vi "Half-H.vi"(8 "error in (no error)":errorcluster, 11 "Node Ptr":T8 format="%.0x") -> (0 "error out":errorcluster)   [LabVIEW 2016, in "DCM System Explorer.lvlib"]
uses:
  DCM System Explorer.lvlib
  <vilib>/NI Veristand/Custom Device API/Custom Device Item Ref.ctl
  <vilib>/Powertrain Controls/Device Drivers/DCM/HH/RT/Setup.ctl
  <vilib>/Powertrain Controls/Device Drivers/DCM/HH/FPGA/Mode.ctl
  <vilib>/Powertrain Controls/Device Drivers/DCM/Rev0/FPGA/Digital Channel.ctl
  <vilib>/Powertrain Controls/Device Drivers/DCM/HH/RT/Angle Control.ctl
  <vilib>/Powertrain Controls/Device Drivers/DCM/HH/RT/Config.ctl
  <vilib>/Powertrain Controls/Device Drivers/DCM/HH/RT/Mode.ctl
  <vilib>/Powertrain Controls/Device Drivers/DCM/HH/RT/ISeq.ctl
  Shared/DCM Properties.vi
  <vilib>/NI Veristand/Custom Device API/Get Item Property (String Array).vi
  Shared/DCM Constants and GUIDs.vi
  <vilib>/NI Veristand/Custom Device API/Set Item Property (String Array).vi
  <vilib>/NI VeriStand/Custom Device API/Custom Device API.lvlib
  DCM Shared.lvlib
  <vilib>/Powertrain Controls/Device Drivers/DCM/HH/RT/DCM - RT - HH.lvlib
  <vilib>/Powertrain Controls/Device Drivers/DCM/Rev0/FPGA/DCM - FPGA.lvlib
  <vilib>/Powertrain Controls/Device Drivers/DCM/HH/FPGA/DCM - FPGA - HH.lvlib
panel:
  in  "Channel Name":string
  in  "Channel Names":string[](array[string])=["", "", "", "", "", "", "", "", "", "", "", ""]
  in  "_Refresh":bool
  in  "_CommandElement":T1={"Mode"=enum."Off", "Digital Input"=enum."Unused", "Polarity"=FALSE, "Frequency [Hz]"=0.0, "Duty Cycle [%]"=0.0, "TDC Offset [CAD]"=0.0, "Window Start [DBTDC]"=0.0, "Window End [DBTDC]"=0.0, "Angles"=[{"Enable"=FALSE, "Location [DBTDC]"=0.0, "Duration [s]"=0.0}, {"Enable"=FALSE, "Location [DBTDC]"=0.0, "Duration [s]"=0.0}, {"Enable"=FALSE, "Location [DBTDC]"=0.0, "Duration [s]"=0.0}, {"Enable"=FALSE, "Location [DBTDC]"=0.0, "Duration [s]"=0.0}], "Skip Fire"=FALSE, "Skip Fire Index"=0} caption="Command Setup" {"Skip Fire Index" max=7; "Angles"."Duration [s]" format="%#_3p"; "Frequency [Hz]" format="%#_3p"}
  in  "_ConfigElement":T5 caption="Channel Configuration" {"ISeq"."Duration [s]" min=0 max=26 format="%#_3p"; "ISeq"."Lower [A]" min=0 max=8 format="%#_3p"; "ISeq"."Upper [A]" min=0 max=8 format="%#_3p"}
  in  "_HH Channels":i32[](listbox) caption="Half-H Channel Summary"
  in  "_Save Changes?":bool
  in  "Command":T1[](array[typedef])=[{"Mode"=enum."Off", "Digital Input"=enum."Unused", "Polarity"=FALSE, "Frequency [Hz]"=0.0, "Duty Cycle [%]"=0.0, "TDC Offset [CAD]"=0.0, "Window Start [DBTDC]"=0.0, "Window End [DBTDC]"=0.0, "Angles"=[{"Enable"=FALSE, "Location [DBTDC]"=0.0, "Duration [s]"=0.0}, {"Enable"=FALSE, "Location [DBTDC]"=0.0, "Duration [s]"=0.0}, {"Enable"=FALSE, "Location [DBTDC]"=0.0, "Duration [s]"=0.0}, {"Enable"=FALSE, "Location [DBTDC]"=0.0, "Duration [s]"=0.0}], "Skip Fire"=FALSE, "Skip Fire Index"=0}, {"Mode"=enum."Off", "Digital Input"=enum."Unused", "Polarity"=FALSE, "Frequency [Hz]"=0.0, "Duty Cycle [%]"=0.0, "TDC Offset [CAD]"=0.0, "Window Start [DBTDC]"=0.0, "Window End [DBTDC]"=0.0, "Angles"=[{"Enable"=FALSE, "Location [DBTDC]"=0.0, "Duration [s]"=0.0}, {"Enable"=FALSE, "Location [DBTDC]"=0.0, "Duration [s]"=0.0}, {"Enable"=FALSE, "Location [DBTDC]"=0.0, "Duration [s]"=0.0}, {"Enable"=FALSE, "Location [DBTDC]"=0.0, "Duration [s]"=0.0}], "Skip Fire"=FALSE, "Skip Fire Index"=0}, {"Mode"=enum."Off", "Digital Input"=enum."Unused", "Polarity"=FALSE, "Frequency [Hz]"=0.0, "Duty Cycle [%]"=0.0, "TDC Offset [CAD]"=0.0, "Window Start [DBTDC]"=0.0, "Window End [DBTDC]"=0.0, "Angles"=[{"Enable"=FALSE, "Location [DBTDC]"=0.0, "Duration [s]"=0.0}, {"Enable"=FALSE, "Location [DBTDC]"=0.0, "Duration [s]"=0.0}, {"Enable"=FALSE, "Location [DBTDC]"=0.0, "Duration [s]"=0.0}, {"Enable"=FALSE, "Location [DBTDC]"=0.0, "Duration [s]"=0.0}], "Skip Fire"=FALSE, "Skip Fire Index"=0}, {"Mode"=enum."Off", "Digital Input"=enum."Unused", "Polarity"=FALSE, "Frequency [Hz]"=0.0, "Duty Cycle [%]"=0.0, "TDC Offset [CAD]"=0.0, "Window Start [DBTDC]"=0.0, "Window End [DBTDC]"=0.0, "Angles"=[{"Enable"=FALSE, "Location [DBTDC]"=0.0, "Duration [s]"=0.0}, {"Enable"=FALSE, "Location [DBTDC]"=0.0, "Duration [s]"=0.0}, {"Enable"=FALSE, "Location [DBTDC]"=0.0, "Duration [s]"=0.0}, {"Enable"=FALSE, "Location [DBTDC]"=0.0, "Duration [s]"=0.0}], "Skip Fire"=FALSE, "Skip Fire Index"=0}, {"Mode"=enum."Off", "Digital Input"=enum."Unused", "Polarity"=FALSE, "Frequency [Hz]"=0.0, "Duty Cycle [%]"=0.0, "TDC Offset [CAD]"=0.0, "Window Start [DBTDC]"=0.0, "Window End [DBTDC]"=0.0, "Angles"=[{"Enable"=FALSE, "Location [DBTDC]"=0.0, "Duration [s]"=0.0}, {"Enable"=FALSE, "Location [DBTDC]"=0.0, "Duration [s]"=0.0}, {"Enable"=FALSE, "Location [DBTDC]"=0.0, "Duration [s]"=0.0}, {"Enable"=FALSE, "Location [DBTDC]"=0.0, "Duration [s]"=0.0}], "Skip Fire"=FALSE, "Skip Fire Index"=0}, {"Mode"=enum."Off", "Digital Input"=enum."Unused", "Polarity"=FALSE, "Frequency [Hz]"=0.0, "Duty Cycle [%]"=0.0, "TDC Offset [CAD]"=0.0, "Window Start [DBTDC]"=0.0, "Window End [DBTDC]"=0.0, "Angles"=[{"Enable"=FALSE, "Location [DBTDC]"=0.0, "Duration [s]"=0.0}, {"Enable"=FALSE, "Location [DBTDC]"=0.0, "Duration [s]"=0.0}, {"Enable"=FALSE, "Location [DBTDC]"=0.0, "Duration [s]"=0.0}, {"Enable"=FALSE, "Location [DBTDC]"=0.0, "Duration [s]"=0.0}], "Skip Fire"=FALSE, "Skip Fire Index"=0}, {"Mode"=enum."Off", "Digital Input"=enum."Unused", "Polarity"=FALSE, "Frequency [Hz]"=0.0, "Duty Cycle [%]"=0.0, "TDC Offset [CAD]"=0.0, "Window Start [DBTDC]"=0.0, "Window End [DBTDC]"=0.0, "Angles"=[{"Enable"=FALSE, "Location [DBTDC]"=0.0, "Duration [s]"=0.0}, {"Enable"=FALSE, "Location [DBTDC]"=0.0, "Duration [s]"=0.0}, {"Enable"=FALSE, "Location [DBTDC]"=0.0, "Duration [s]"=0.0}, {"Enable"=FALSE, "Location [DBTDC]"=0.0, "Duration [s]"=0.0}], "Skip Fire"=FALSE, "Skip Fire Index"=0}, {"Mode"=enum."Off", "Digital Input"=enum."Unused", "Polarity"=FALSE, "Frequency [Hz]"=0.0, "Duty Cycle [%]"=0.0, "TDC Offset [CAD]"=0.0, "Window Start [DBTDC]"=0.0, "Window End [DBTDC]"=0.0, "Angles"=[{"Enable"=FALSE, "Location [DBTDC]"=0.0, "Duration [s]"=0.0}, {"Enable"=FALSE, "Location [DBTDC]"=0.0, "Duration [s]"=0.0}, {"Enable"=FALSE, "Location [DBTDC]"=0.0, "Duration [s]"=0.0}, {"Enable"=FALSE, "Location [DBTDC]"=0.0, "Duration [s]"=0.0}], "Skip Fire"=FALSE, "Skip Fire Index"=0}] {"Skip Fire Index" max=7; "Angles"."Duration [s]" format="%#_3p"; "Frequency [Hz]" format="%#_3p"}
  in  "Config":T5[](array[typedef])=[{"Mode"=enum."Off", "IO Lock State"=FALSE, "Phase 1 FP"=FALSE, "Fault Clear"=FALSE, "ISeq"=[]}, {"Mode"=enum."Off", "IO Lock State"=FALSE, "Phase 1 FP"=FALSE, "Fault Clear"=FALSE, "ISeq"=[]}, {"Mode"=enum."Off", "IO Lock State"=FALSE, "Phase 1 FP"=FALSE, "Fault Clear"=FALSE, "ISeq"=[]}, {"Mode"=enum."Off", "IO Lock State"=FALSE, "Phase 1 FP"=FALSE, "Fault Clear"=FALSE, "ISeq"=[]}, {"Mode"=enum."Off", "IO Lock State"=FALSE, "Phase 1 FP"=FALSE, "Fault Clear"=FALSE, "ISeq"=[]}, {"Mode"=enum."Off", "IO Lock State"=FALSE, "Phase 1 FP"=FALSE, "Fault Clear"=FALSE, "ISeq"=[]}, {"Mode"=enum."Off", "IO Lock State"=FALSE, "Phase 1 FP"=FALSE, "Fault Clear"=FALSE, "ISeq"=[]}, {"Mode"=enum."Off", "IO Lock State"=FALSE, "Phase 1 FP"=FALSE, "Fault Clear"=FALSE, "ISeq"=[]}] {"ISeq"."Duration [s]" min=0 max=26 format="%#_3p"; "ISeq"."Lower [A]" min=0 max=8 format="%#_3p"; "ISeq"."Upper [A]" min=0 max=8 format="%#_3p"}
  in  "Header":cluster{"Section Name":string}={"Section Name"="Half-H Drive Initial Settings"}
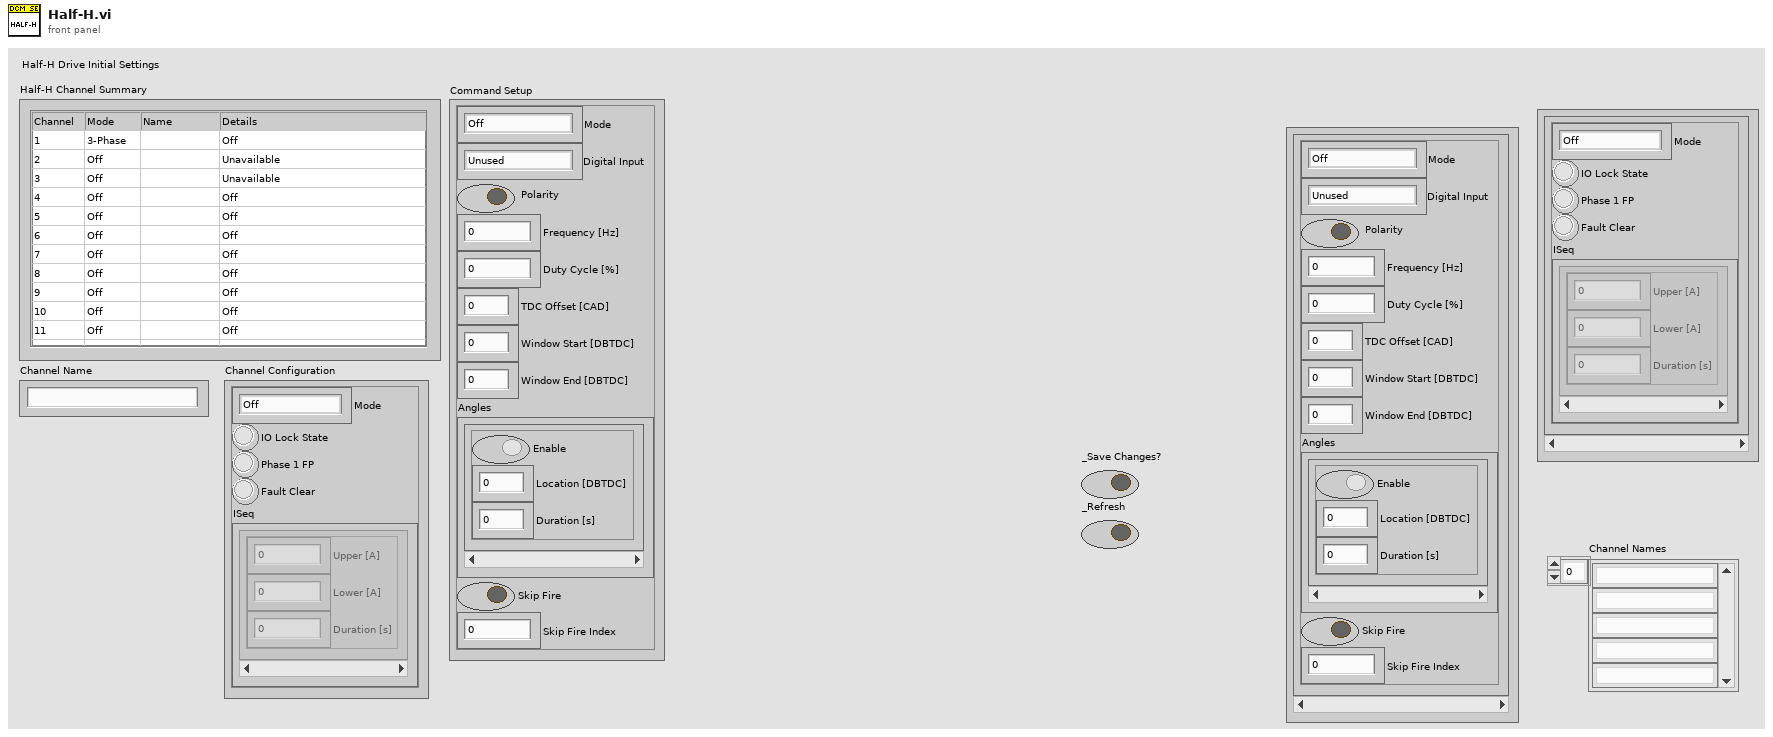
[diagram p1: front panel]
types:
  T1 = typedef "DCM - RT - HH.lvlib/Setup.ctl" = cluster{"Mode":T2, "Digital Input":T3, "Polarity":bool, "Frequency [Hz]":sgl, "Duty Cycle [%]":sgl, "TDC Offset [CAD]":sgl, "Window Start [DBTDC]":sgl, "Window End [DBTDC]":sgl, "Angles":T4[], "Skip Fire":bool, "Skip Fire Index":u8}
  T2 = typedef "DCM - FPGA - HH.lvlib/Mode.ctl" = enum8{"Off", "Direct", "Pulse Width Modulation", "Engine Position Tracking"}
  T3 = typedef "DCM - FPGA.lvlib/Digital Channel.ctl" = enum8{"Unused", "User OS", "Diff IO 1", "Diff IO 2", "Diff IO 3", "Diff IO 4", "Diff IO 5", "Diff IO 6", "Diff IO 7", "Diff IO 8", "Aux 1", "Aux 2", "Aux 3", "Aux 4", "Aux 5", "Aux 6", "Aux 7", "Aux 8", "Aux 9", "Aux 10", "Aux 11", "Aux 12", "Aux 13", "Aux 14", "Aux 15", "Aux 16"}
  T4 = typedef "DCM - RT - HH.lvlib/Angle Control.ctl" = cluster{"Enable":bool, "Location [DBTDC]":sgl, "Duration [s]":sgl}
  T5 = typedef "DCM - RT - HH.lvlib/Config.ctl" = cluster{"Mode":T6, "IO Lock State":bool, "Phase 1 FP":bool, "Fault Clear":bool, "ISeq":T7[]}
  T6 = typedef "DCM - RT - HH.lvlib/Mode.ctl" = enum16{"Off", "Lowside", "Highside", "PFI", "Full H", "3-Phase"}
  T7 = typedef "DCM - RT - HH.lvlib/ISeq.ctl" = cluster{"Upper [A]":sgl, "Lower [A]":sgl, "Duration [s]":sgl}
  T8 = typedef "Custom Device API.lvlib/Custom Device Item Ref.ctl" = u64
  T9 = typedef "Custom Device API.lvlib/Custom Device Commands.ctl" = enum16{"Default", "Item renamed", "Shutdown", "Dynamic button pressed"}
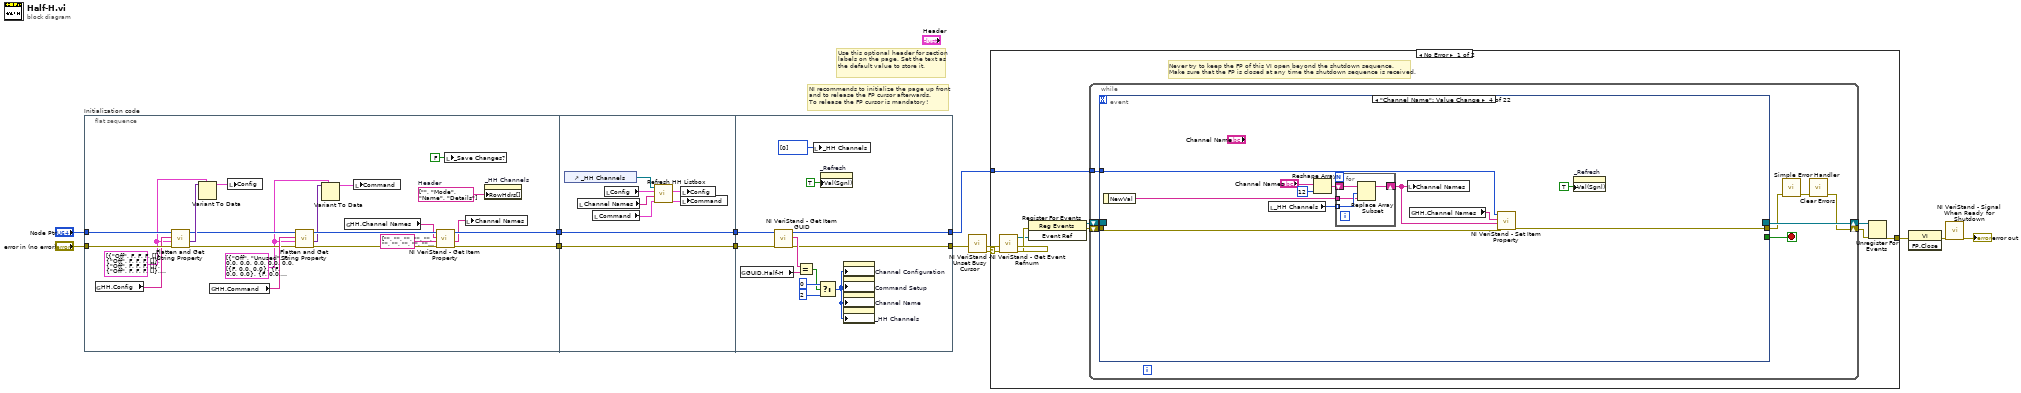
[diagram p0: block diagram]
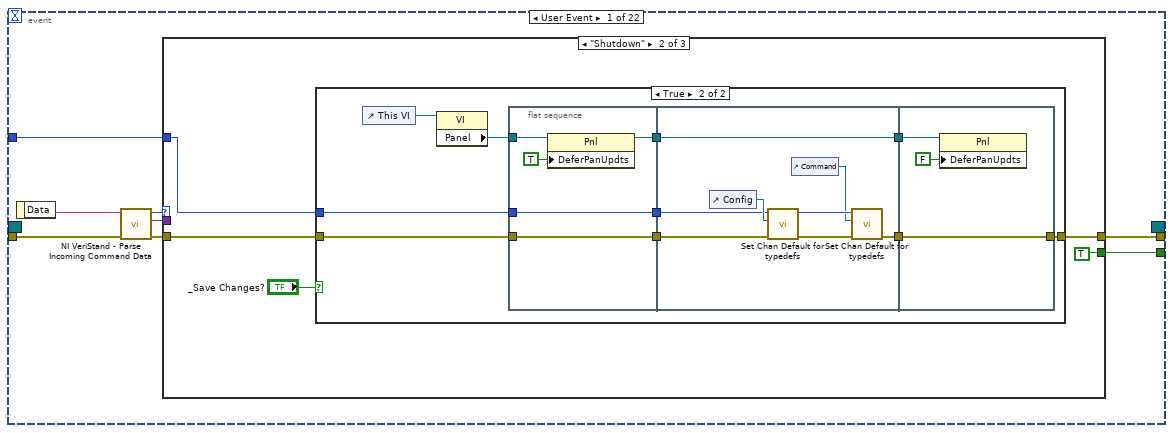
[diagram p2: hidden frame]
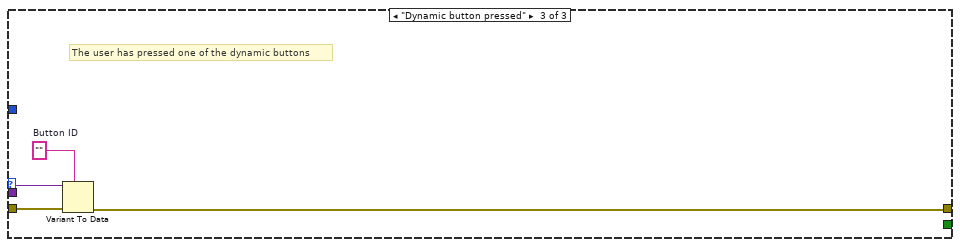
[diagram p5: hidden frame]
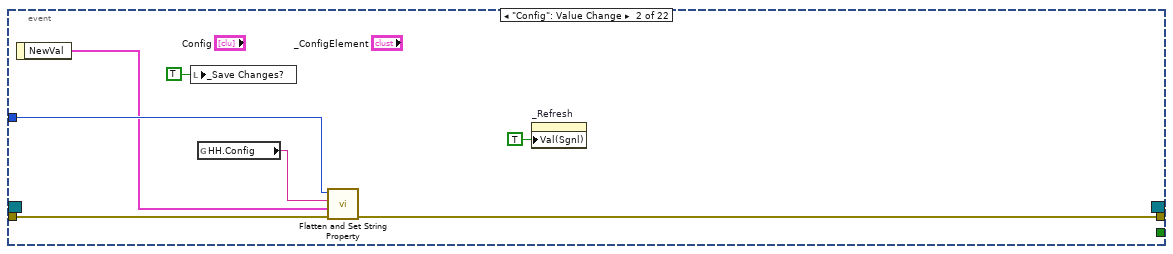
[diagram p6: hidden frame]
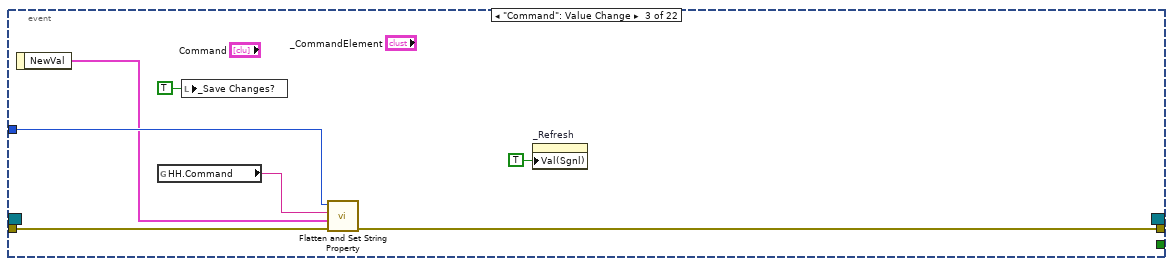
[diagram p7: hidden frame]
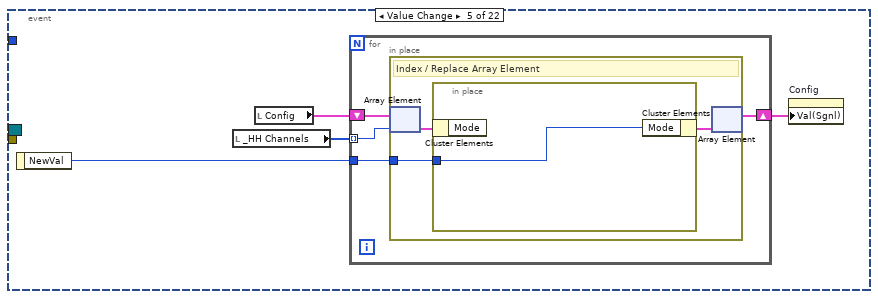
[diagram p8: hidden frame]
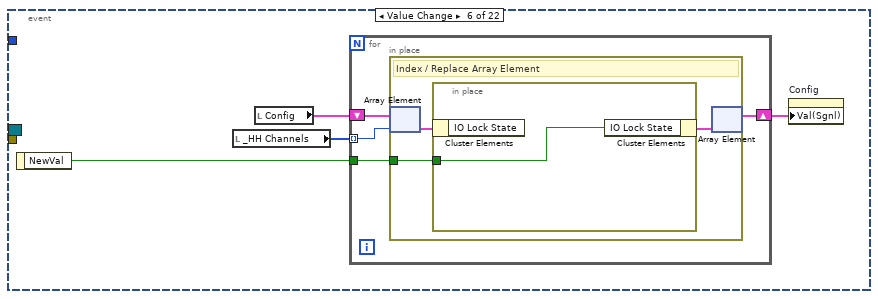
[diagram p9: hidden frame]
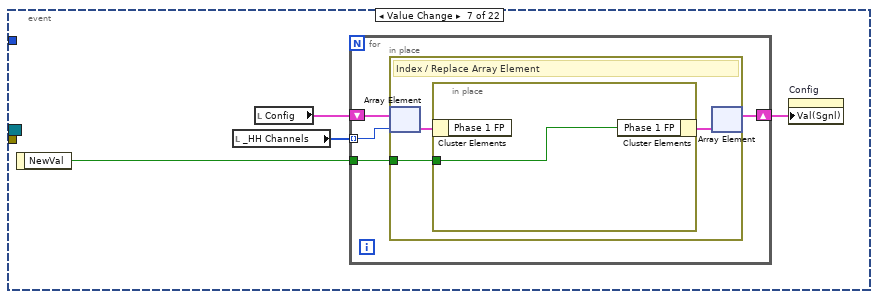
[diagram p10: hidden frame]
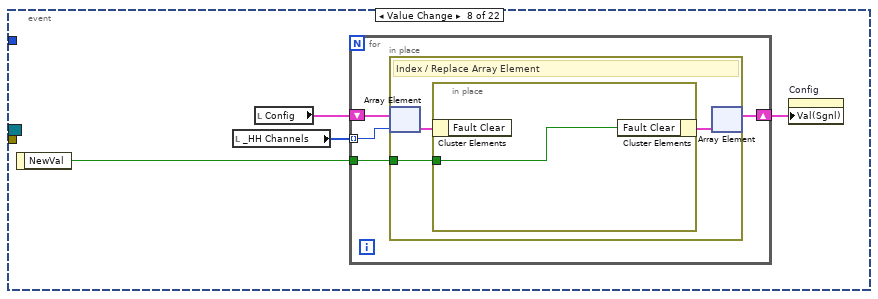
[diagram p11: hidden frame]
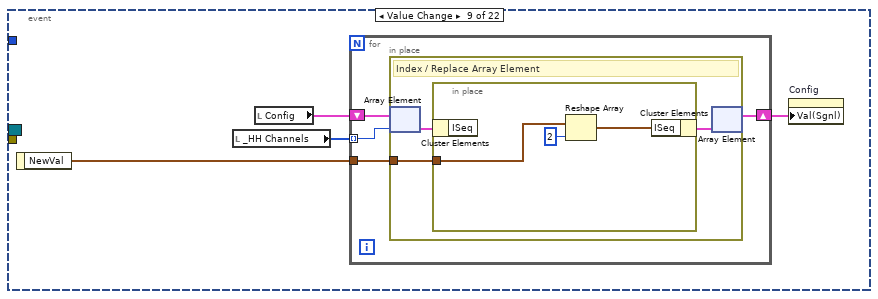
[diagram p12: hidden frame]
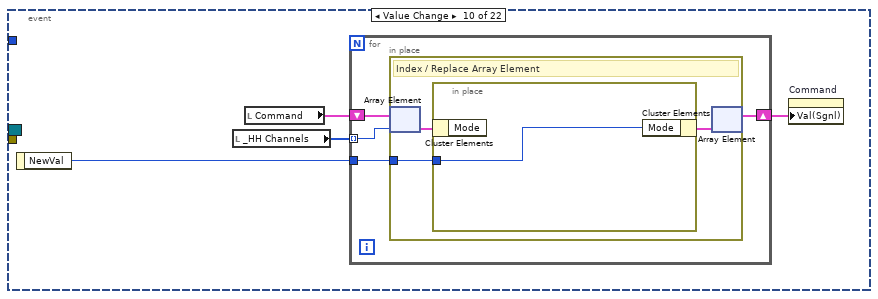
[diagram p13: hidden frame]
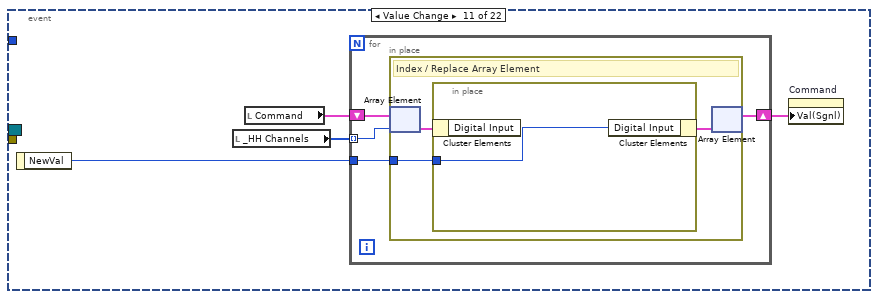
[diagram p14: hidden frame]
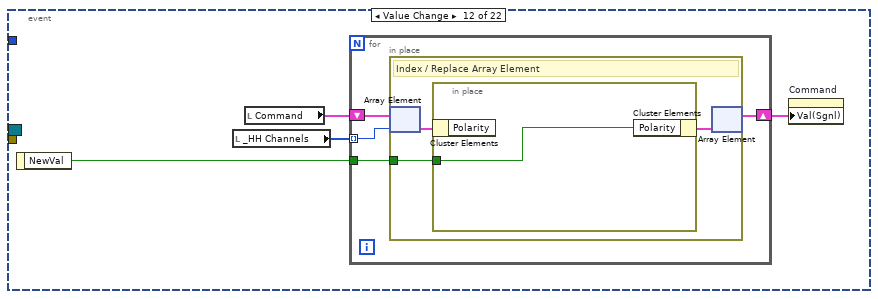
[diagram p15: hidden frame]
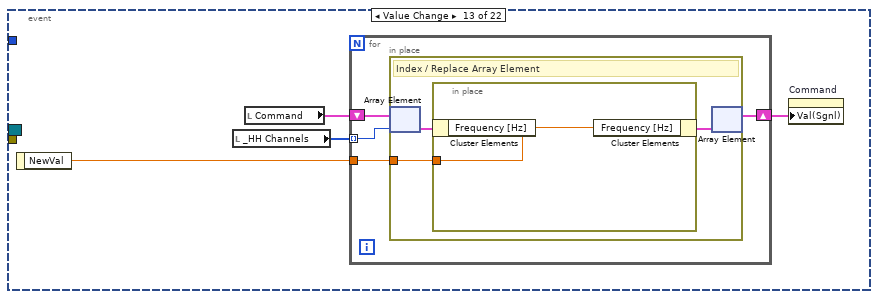
[diagram p16: hidden frame]
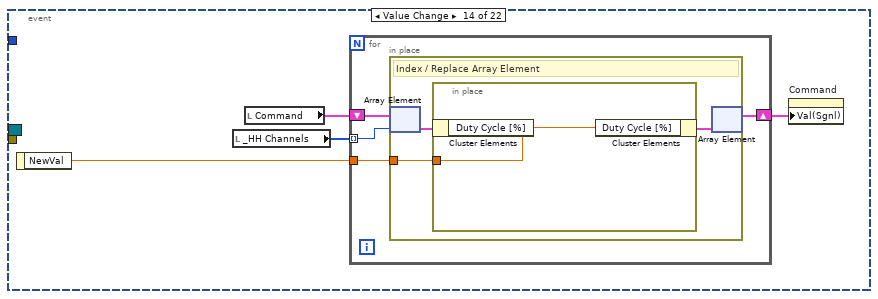
[diagram p17: hidden frame]
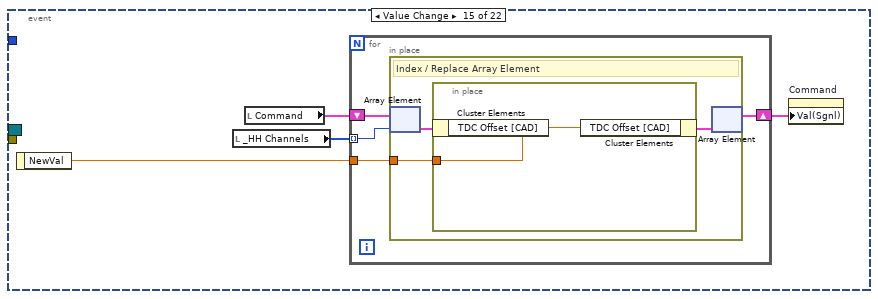
[diagram p18: hidden frame]
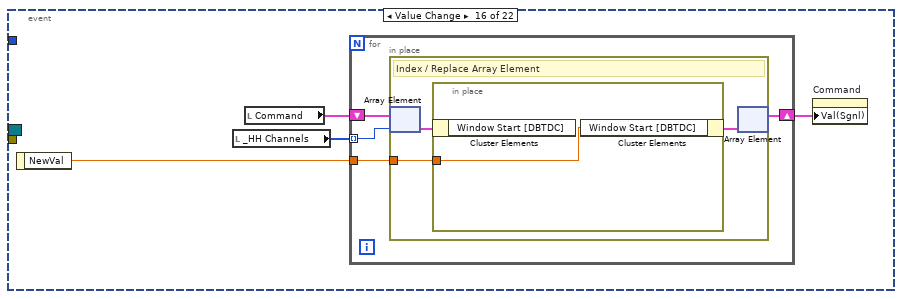
[diagram p19: hidden frame]
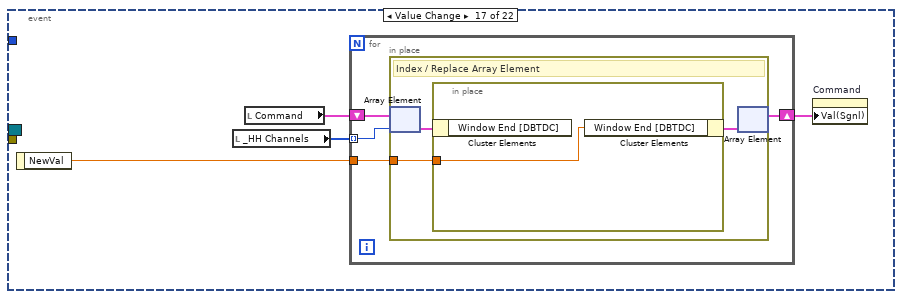
[diagram p20: hidden frame]
diagram:
  # "Use this optional header for section labels on the page. Set the text as the default value to store it."
  # "NI recommends to initialize the page up front\nand to release the FP cursor afterwards.\nTo release the FP cursor is mandatory!"
  n1 = flat-sequence "Initialization code" {
    tunnel: "Node Ptr" -> [w30]
    tunnel: "error in (no error)" -> [w31]
    tunnel: [w14] -> w5
    tunnel: [w15] -> w4
    tunnel: w4 -> [w40]
    tunnel: w5 -> [w41]
    tunnel: [w41] -> w3
    tunnel: [w40] -> w2
    tunnel: [w45] -> w1
    tunnel: [w44] -> w6
    tunnel: w3 -> [w46]
    tunnel: w2 -> [w47]
    frame #0 {
      w16 = string[] ["", "Mode", "Name", "Details"]  # Header
      w21 = T5[] [{"Mode"=enum."Off", "IO Lock State"=FALSE, "Phase 1 FP"=FALSE, "Fault Clear"=FALSE, "ISeq"=[]}, {"Mode"=enum."Off", "IO Lock State"=FALSE, "Phase 1 FP"=FALSE, "Fault Clear"=FALSE, "ISeq"=[]}, {"Mode"=enum."Off", "IO Lock State"=FALSE, "Phase 1 FP"=FALSE, "Fault Clear"=FALSE, "ISeq"=[]}, {"Mode"=enum."Off", "IO Lock State"=FALSE, "Phase 1 FP"=FALSE, "Fault Clear"=FALSE, "ISeq"=[]}, {"Mode"=enum."Off", "IO Lock State"=FALSE, "Phase 1 FP"=FALSE, "Fault Clear"=FALSE, "ISeq"=[]}, {"Mode"=enum."Off", "IO Lock State"=FALSE, "Phase 1 FP"=FALSE, "Fault Clear"=FALSE, "ISeq"=[]}, {"Mode"=enum."Off", "IO Lock State"=FALSE, "Phase 1 FP"=FALSE, "Fault Clear"=FALSE, "ISeq"=[]}, {"Mode"=enum."Off", "IO Lock State"=FALSE, "Phase 1 FP"=FALSE, "Fault Clear"=FALSE, "ISeq"=[]}, {"Mode"=enum."Off", "IO Lock State"=FALSE, "Phase 1 FP"=FALSE, "Fault Clear"=FALSE, "ISeq"=[]}, {"Mode"=enum."Off", "IO Lock State"=FALSE, "Phase 1 FP"=FALSE, "Fault Clear"=FALSE, "ISeq"=[]}, {"Mode"=enum."Off", "IO Lock State"=FALSE, "Phase 1 FP"=FALSE, "Fault Clear"=FALSE, "ISeq"=[]}, {"Mode"=enum."Off", "IO Lock State"=FALSE, "Phase 1 FP"=FALSE, "Fault Clear"=FALSE, "ISeq"=[]}] ("HH Config")
      w22 = T1[] [{"Mode"=enum."Off", "Digital Input"=enum."Unused", "Polarity"=FALSE, "Frequency [Hz]"=0.0, "Duty Cycle [%]"=0.0, "TDC Offset [CAD]"=0.0, "Window Start [DBTDC]"=0.0, "Window End [DBTDC]"=0.0, "Angles"=[{"Enable"=FALSE, "Location [DBTDC]"=0.0, "Duration [s]"=0.0}, {"Enable"=FALSE, "Location [DBTDC]"=0.0, "Duration [s]"=0.0}, {"Enable"=FALSE, "Location [DBTDC]"=0.0, "Duration [s]"=0.0}, {"Enable"=FALSE, "Location [DBTDC]"=0.0, "Duration [s]"=0.0}], "Skip Fire"=FALSE, "Skip Fire Index"=0}, {"Mode"=enum."Off", "Digital Input"=enum."Unused", "Polarity"=FALSE, "Frequency [Hz]"=0.0, "Duty Cycle [%]"=0.0, "TDC Offset [CAD]"=0.0, "Window Start [DBTDC]"=0.0, "Window End [DBTDC]"=0.0, "Angles"=[{"Enable"=FALSE, "Location [DBTDC]"=0.0, "Duration [s]"=0.0}, {"Enable"=FALSE, "Location [DBTDC]"=0.0, "Duration [s]"=0.0}, {"Enable"=FALSE, "Location [DBTDC]"=0.0, "Duration [s]"=0.0}, {"Enable"=FALSE, "Location [DBTDC]"=0.0, "Duration [s]"=0.0}], "Skip Fire"=FALSE, "Skip Fire Index"=0}, {"Mode"=enum."Off", "Digital Input"=enum."Unused", "Polarity"=FALSE, "Frequency [Hz]"=0.0, "Duty Cycle [%]"=0.0, "TDC Offset [CAD]"=0.0, "Window Start [DBTDC]"=0.0, "Window End [DBTDC]"=0.0, "Angles"=[{"Enable"=FALSE, "Location [DBTDC]"=0.0, "Duration [s]"=0.0}, {"Enable"=FALSE, "Location [DBTDC]"=0.0, "Duration [s]"=0.0}, {"Enable"=FALSE, "Location [DBTDC]"=0.0, "Duration [s]"=0.0}, {"Enable"=FALSE, "Location [DBTDC]"=0.0, "Duration [s]"=0.0}], "Skip Fire"=FALSE, "Skip Fire Index"=0}, {"Mode"=enum."Off", "Digital Input"=enum."Unused", "Polarity"=FALSE, "Frequency [Hz]"=0.0, "Duty Cycle [%]"=0.0, "TDC Offset [CAD]"=0.0, "Window Start [DBTDC]"=0.0, "Window End [DBTDC]"=0.0, "Angles"=[{"Enable"=FALSE, "Location [DBTDC]"=0.0, "Duration [s]"=0.0}, {"Enable"=FALSE, "Location [DBTDC]"=0.0, "Duration [s]"=0.0}, {"Enable"=FALSE, "Location [DBTDC]"=0.0, "Duration [s]"=0.0}, {"Enable"=FALSE, "Location [DBTDC]"=0.0, "Duration [s]"=0.0}], "Skip Fire"=FALSE, "Skip Fire Index"=0}, {"Mode"=enum."Off", "Digital Input"=enum."Unused", "Polarity"=FALSE, "Frequency [Hz]"=0.0, "Duty Cycle [%]"=0.0, "TDC Offset [CAD]"=0.0, "Window Start [DBTDC]"=0.0, "Window End [DBTDC]"=0.0, "Angles"=[{"Enable"=FALSE, "Location [DBTDC]"=0.0, "Duration [s]"=0.0}, {"Enable"=FALSE, "Location [DBTDC]"=0.0, "Duration [s]"=0.0}, {"Enable"=FALSE, "Location [DBTDC]"=0.0, "Duration [s]"=0.0}, {"Enable"=FALSE, "Location [DBTDC]"=0.0, "Duration [s]"=0.0}], "Skip Fire"=FALSE, "Skip Fire Index"=0}, {"Mode"=enum."Off", "Digital Input"=enum."Unused", "Polarity"=FALSE, "Frequency [Hz]"=0.0, "Duty Cycle [%]"=0.0, "TDC Offset [CAD]"=0.0, "Window Start [DBTDC]"=0.0, "Window End [DBTDC]"=0.0, "Angles"=[{"Enable"=FALSE, "Location [DBTDC]"=0.0, "Duration [s]"=0.0}, {"Enable"=FALSE, "Location [DBTDC]"=0.0, "Duration [s]"=0.0}, {"Enable"=FALSE, "Location [DBTDC]"=0.0, "Duration [s]"=0.0}, {"Enable"=FALSE, "Location [DBTDC]"=0.0, "Duration [s]"=0.0}], "Skip Fire"=FALSE, "Skip Fire Index"=0}, {"Mode"=enum."Off", "Digital Input"=enum."Unused", "Polarity"=FALSE, "Frequency [Hz]"=0.0, "Duty Cycle [%]"=0.0, "TDC Offset [CAD]"=0.0, "Window Start [DBTDC]"=0.0, "Window End [DBTDC]"=0.0, "Angles"=[{"Enable"=FALSE, "Location [DBTDC]"=0.0, "Duration [s]"=0.0}, {"Enable"=FALSE, "Location [DBTDC]"=0.0, "Duration [s]"=0.0}, {"Enable"=FALSE, "Location [DBTDC]"=0.0, "Duration [s]"=0.0}, {"Enable"=FALSE, "Location [DBTDC]"=0.0, "Duration [s]"=0.0}], "Skip Fire"=FALSE, "Skip Fire Index"=0}, {"Mode"=enum."Off", "Digital Input"=enum."Unused", "Polarity"=FALSE, "Frequency [Hz]"=0.0, "Duty Cycle [%]"=0.0, "TDC Offset [CAD]"=0.0, "Window Start [DBTDC]"=0.0, "Window End [DBTDC]"=0.0, "Angles"=[{"Enable"=FALSE, "Location [DBTDC]"=0.0, "Duration [s]"=0.0}, {"Enable"=FALSE, "Location [DBTDC]"=0.0, "Duration [s]"=0.0}, {"Enable"=FALSE, "Location [DBTDC]"=0.0, "Duration [s]"=0.0}, {"Enable"=FALSE, "Location [DBTDC]"=0.0, "Duration [s]"=0.0}], "Skip Fire"=FALSE, "Skip Fire Index"=0}, {"Mode"=enum."Off", "Digital Input"=enum."Unused", "Polarity"=FALSE, "Frequency [Hz]"=0.0, "Duty Cycle [%]"=0.0, "TDC Offset [CAD]"=0.0, "Window Start [DBTDC]"=0.0, "Window End [DBTDC]"=0.0, "Angles"=[{"Enable"=FALSE, "Location [DBTDC]"=0.0, "Duration [s]"=0.0}, {"Enable"=FALSE, "Location [DBTDC]"=0.0, "Duration [s]"=0.0}, {"Enable"=FALSE, "Location [DBTDC]"=0.0, "Duration [s]"=0.0}, {"Enable"=FALSE, "Location [DBTDC]"=0.0, "Duration [s]"=0.0}], "Skip Fire"=FALSE, "Skip Fire Index"=0}, {"Mode"=enum."Off", "Digital Input"=enum."Unused", "Polarity"=FALSE, "Frequency [Hz]"=0.0, "Duty Cycle [%]"=0.0, "TDC Offset [CAD]"=0.0, "Window Start [DBTDC]"=0.0, "Window End [DBTDC]"=0.0, "Angles"=[{"Enable"=FALSE, "Location [DBTDC]"=0.0, "Duration [s]"=0.0}, {"Enable"=FALSE, "Location [DBTDC]"=0.0, "Duration [s]"=0.0}, {"Enable"=FALSE, "Location [DBTDC]"=0.0, "Duration [s]"=0.0}, {"Enable"=FALSE, "Location [DBTDC]"=0.0, "Duration [s]"=0.0}], "Skip Fire"=FALSE, "Skip Fire Index"=0}, {"Mode"=enum."Off", "Digital Input"=enum."Unused", "Polarity"=FALSE, "Frequency [Hz]"=0.0, "Duty Cycle [%]"=0.0, "TDC Offset [CAD]"=0.0, "Window Start [DBTDC]"=0.0, "Window End [DBTDC]"=0.0, "Angles"=[{"Enable"=FALSE, "Location [DBTDC]"=0.0, "Duration [s]"=0.0}, {"Enable"=FALSE, "Location [DBTDC]"=0.0, "Duration [s]"=0.0}, {"Enable"=FALSE, "Location [DBTDC]"=0.0, "Duration [s]"=0.0}, {"Enable"=FALSE, "Location [DBTDC]"=0.0, "Duration [s]"=0.0}], "Skip Fire"=FALSE, "Skip Fire Index"=0}, {"Mode"=enum."Off", "Digital Input"=enum."Unused", "Polarity"=FALSE, "Frequency [Hz]"=0.0, "Duty Cycle [%]"=0.0, "TDC Offset [CAD]"=0.0, "Window Start [DBTDC]"=0.0, "Window End [DBTDC]"=0.0, "Angles"=[{"Enable"=FALSE, "Location [DBTDC]"=0.0, "Duration [s]"=0.0}, {"Enable"=FALSE, "Location [DBTDC]"=0.0, "Duration [s]"=0.0}, {"Enable"=FALSE, "Location [DBTDC]"=0.0, "Duration [s]"=0.0}, {"Enable"=FALSE, "Location [DBTDC]"=0.0, "Duration [s]"=0.0}], "Skip Fire"=FALSE, "Skip Fire Index"=0}] ("Half-H Command")
      n2 = global read "DCM Properties.vi" "HH.Config"() -> (w27:string)
      n3 = call "Flatten and Get String Property.vi"("error in (no error)"=w31, "Default Value"=w21, "Property Name"=w27, "Section Ref in"=w30) -> ("error out"=w24:errorcluster, "Value"=w29:variant, "Section Ref out"=w25:T8)  [unwired: 5 in]
      n4 = Variant To Data(type=w21, Variant=w29) -> (data=w23:T5[])  [unwired: 1 in, 1 out]
      n5 = global read "DCM Properties.vi" "HH.Command"() -> (w26:string)
      n6 = local write "Config"(w23) -> ()
      n7 = call "Flatten and Get String Property.vi"("error in (no error)"=w24, "Default Value"=w22, "Property Name"=w26, "Section Ref in"=w25) -> ("error out"=w32:errorcluster, "Value"=w28:variant, "Section Ref out"=w33:T8)  [unwired: 5 in]
      n8 = Variant To Data(type=w22, Variant=w28) -> (data=w20:T1[])  [unwired: 1 in, 1 out]
      n9 = global read "DCM Properties.vi" "HH.Channel Names"() -> (w18:string)
      n10 = local write "Command"(w20) -> ()
      n11 = call-poly <vilib>:"NI VeriStand - Get Item Property.vi"("error in (no error)"=w32, "Default Value"=string[] ["", "", "", "", "", "", "", "", "", "", "", ""], "Property Name"=w18, "Item Ref in"=w33) -> ("error out"=w14:errorcluster, "Value"=w13:string[], "Item Ref out"=w15:T8)  [unwired: 4 in, 1 out]
      n12 = local write "_Save Changes?"(FALSE ("_Save Changes?")) -> ()
      n13 = local write "Channel Names"(w13) -> ()
      n14 = property on="_HH Channels" class="MCListbox (strict)"("RowHdrs[]"=w16) -> ()  [unwired: 2 in, 2 out]
    }
    frame #1 {
      n15 = control-ref of="_HH Channels"() -> (w39:refnum<vi>)
      n16 = local read "Channel Names"() -> (w37:string[])
      n17 = local read "Command"() -> (w35:T1[])
      n18 = local read "Config"() -> (w38:T5[])
      n19 = call "Refresh HH Listbox.vi"("Command"=w35, "Names"=w37, "Config"=w38, "_Listbox"=w39) -> ("Command out"=w34:T1[], "Config out"=w36:T5[])  [unwired: 6 in]
      n20 = local write "Config"(w36) -> ()
      n21 = local write "Command"(w34) -> ()
    }
    frame #2 {
      n22 = global read "DCM Constants and GUIDs.vi" "GUID.Half-H"() -> (w49:string)
      n23 = call <vilib>:"NI VeriStand - Get Item GUID.vi"("error in (no error)"=w46, "Item Ref in"=w47) -> ("error out"=w44:errorcluster, "GUID"=w50:string, "Item Ref out"=w45:T8)  [unwired: 7 in]
      n24 = Equal?(x=w50, y=w49) -> (x = y?=w48:bool)
      n25 = local write "_HH Channels"(i32[] [0] ("_HH Channels")) -> ()
      n26 = Select(t=0, s=w48, f=2) -> (s? t:f=w53:i32)
      n27 = property on="_Refresh" class="Bool (strict)"("Val(Sgnl)"=TRUE ("Value (Signaling)")) -> ()  [unwired: 2 in, 2 out]
      n28 = property on="Channel Configuration" class="Clust (strict)"("DisabledEnum"=w53) -> ()  [unwired: 2 in, 2 out]
      n29 = property on="Command Setup" class="Clust (strict)"("DisabledEnum"=w53) -> ()  [unwired: 2 in, 2 out]
      n30 = property on="Channel Name" class="Str"("DisabledEnum"=w53) -> ()  [unwired: 2 in, 2 out]
      n31 = property on="_HH Channels" class="MCListbox (strict)"("DisabledEnum"=w53) -> ()  [unwired: 2 in, 2 out]
    }
  }
  n32 = call <vilib>:"NI VeriStand - Unset Busy Cursor.vi"("error in (no error)"=w6) -> ("error out"=w9:errorcluster)  [unwired: 10 out]
  n33 = case shown="No Error" w9 {
    selector: w9 -> [w54 w358]
    tunnel: [w59 w356] -> w12
    tunnel: w1 -> [w55 _]
    frame No Error {
      # "Never try to keep the FP of this VI open beyond the shutdown sequence.\nMake sure that the FP is closed at any time the shutdown sequence is received."
      n34 = call <vilib>:"NI VeriStand - Get Event Refnum.vi"("error in (no error)"=w54) -> ("error out"=w62:errorcluster, "Event Ref"=w58:refnum<user-event>)  [unwired: 9 out]
      n35 = register-events(error in=w62, w58) -> (reference out=w56:refnum<event-registration>, error out=w57:errorcluster)  [unwired: 1 in]
      n36 = while {
        tunnel: w55 -> [w66]
        shift-right: [w63] -> w60
        shift-left: w57 -> [w69]
        shift-right: [w70] -> w61
        shift-left: w56 -> [w68]
        stop <- w67 stop-if-true
        n37 = event shown="[3] \"Channel Name\": Value Change" {
          selector: w68 -> [_ _ _ _ _ _ _ _ _ _ _ _ _ _ _ _ _ _ _ _ _ _]
          dyn-events: [_ _ _ _ _ _ _ _ _ _ _ _ _ _ _ _ _ _ _ _ _ _] -> w70
          timeout: _ -> [_ _ _ _ _ _ _ _ _ _ _ _ _ _ _ _ _ _ _ _ _ _]
          tunnel: w69 -> [w78 w122 w129 w140 _ _ _ _ _ _ _ _ _ _ _ _ _ _ _ _ _ _]
          tunnel: [w74 _ _ _ _ _ _ _ _ _ _ _ _ _ _ _ _ _ _ _ _ _] -> w67
          tunnel: [w73 w121 w128 w139 _ _ _ _ _ _ _ _ _ _ _ _ _ _ _ _ _ _] -> w65
          tunnel: w66 -> [w72 w120 w127 w138 _ _ _ _ _ _ _ _ _ _ _ _ _ _ _ _ _ _]
          event User Event {
            n38 = event-data() -> ("Data"=w77:string)  [unwired: 1 out]
            n39 = call <vilib>:"NI VeriStand - Parse Incoming Command Data.vi"("error in (no error)"=w78, "Incoming data"=w77) -> ("error out"=w76:errorcluster, "Outgoing data"=w71:variant, "Action"=w75:T9)  [unwired: 7 out]
            n40 = case shown="\"Shutdown\"" w75 {
              tunnel: w76 -> [w79 w82 w115]
              tunnel: [_ TRUE _] -> w74
              tunnel: [w79 w81 w112] -> w73
              tunnel: w72 -> [_ w83 _]
              tunnel: w71 -> [_ _ w114]
              frame "Default", Default {
              }
              frame "Shutdown" {
                n41 = case shown="True" "_Save Changes?" {
                  tunnel: w83 -> [_ w90]
                  tunnel: w82 -> [w85 w89]
                  tunnel: [w85 w88] -> w81
                  frame False {
                  }
                  frame True {
                    n42 = control-ref of="This VI"() -> (w87:refnum<vi>)
                    n43 = property class="VI"(reference=w87) -> ("Panel"=w86:refnum<vi>)  [unwired: 1 in, 2 out]
                    n44 = flat-sequence {
                      tunnel: w89 -> [w99]
                      tunnel: w90 -> [w100]
                      tunnel: [w100] -> w95
                      tunnel: [w99] -> w94
                      tunnel: w86 -> [w98]
                      tunnel: [w96] -> w93
                      tunnel: w95 -> [w104]
                      tunnel: w94 -> [w103]
                      tunnel: [w102] -> w92
                      tunnel: [w101] -> w91
                      tunnel: w93 -> [w101]
                      tunnel: [w111] -> w88
                      tunnel: w92 -> [w111]
                      tunnel: w91 -> [w109]
                      frame #0 {
                        n45 = property class="Pnl"(reference=w98, "DeferPanUpdts"=TRUE ("Defer Panel Updates")) -> (reference out=w96:refnum<vi>)  [unwired: 1 in, 1 out]
                      }
                      frame #1 {
                        n46 = control-ref of="Config"() -> (w106:refnum<vi>)
                        n47 = call "Set Chan Default for typedefs.vi"("error in"=w103, "Ctl Ref"=w106, "Section Ref in"=w104) -> ("error out"=w107:errorcluster, "Section Ref out"=w108:T8)  [unwired: 7 in]
                        n48 = control-ref of="Command"() -> (w105:refnum<vi>)
                        n49 = call "Set Chan Default for typedefs.vi"("error in"=w107, "Ctl Ref"=w105, "Section Ref in"=w108) -> ("error out"=w102:errorcluster)  [unwired: 7 in, 1 out]
                      }
                      frame #2 {
                        n50 = property class="Pnl"(reference=w109, "DeferPanUpdts"=FALSE ("Defer Panel Updates")) -> ()  [unwired: 1 in, 2 out]
                      }
                    }
                  }
                }
              }
              frame "Dynamic button pressed" {
                w113 = ""  # Button ID
                # "The user has pressed one of the dynamic buttons"
                n51 = Variant To Data(error in=w115, type=w113, Variant=w114) -> (error out=w112:errorcluster)  [unwired: 1 out]
              }
            }
          }
          event "Config": Value Change {
            n52 = event-data() -> ("NewVal"=w117:T5[])  [unwired: 1 out]
            n53 = local write "_Save Changes?"(TRUE ("_Save Changes?")) -> ()
            n54 = global read "DCM Properties.vi" "HH.Config"() -> (w119:string)
            n55 = call "Flatten and Set String Property.vi"("error in (no error)"=w122, "Value"=w117, "Property Name"=w119, "Section Ref in"=w120) -> ("error out"=w121:errorcluster)  [unwired: 6 in, 1 out]
            n56 = property on="_Refresh" class="Bool (strict)"("Val(Sgnl)"=TRUE ("Value (Signaling)")) -> ()  [unwired: 2 in, 2 out]
          }
          event "Command": Value Change {
            n57 = event-data() -> ("NewVal"=w124:T1[])  [unwired: 1 out]
            n58 = global read "DCM Properties.vi" "HH.Command"() -> (w126:string)
            n59 = local write "_Save Changes?"(TRUE ("_Save Changes?")) -> ()
            n60 = call "Flatten and Set String Property.vi"("error in (no error)"=w129, "Value"=w124, "Property Name"=w126, "Section Ref in"=w127) -> ("error out"=w128:errorcluster)  [unwired: 6 in, 1 out]
            n61 = property on="_Refresh" class="Bool (strict)"("Val(Sgnl)"=TRUE ("Value (Signaling)")) -> ()  [unwired: 2 in, 2 out]
          }
          event "Channel Name": Value Change {
            n62 = event-data() -> ("NewVal"=w133:string)  [unwired: 1 out]
            n63 = local read "_HH Channels"() -> (w134:i32[])
            n64 = Reshape Array("Channel Names", 12 ("dimension size")) -> (w136:string[])
            n65 = for {
              tunnel: w134 -> [w142] mode=indexing
              shift-right: [w143] -> w131
              shift-left: w136 -> [w144]
              tunnel: w133 -> [w141]
              n66 = Replace Array Subset(array=w144, new element=w141, index=w142) -> (w143:string[])
            }
            n67 = local write "Channel Names"(w131) -> ()
            n68 = global read "DCM Properties.vi" "HH.Channel Names"() -> (w137:string)
            n69 = call-poly <vilib>:"NI VeriStand - Set Item Property.vi"("error in (no error)"=w140, "Value"=w131, "Property Name"=w137, "Item Ref in"=w138) -> ("error out"=w139:errorcluster)  [unwired: 5 in, 2 out]
            n70 = property on="_Refresh" class="Bool (strict)"("Val(Sgnl)"=TRUE ("Value (Signaling)")) -> ()  [unwired: 2 in, 2 out]
          }
          event Value Change {
            n71 = event-data() -> ("NewVal"=w148:T6)  [unwired: 1 out]
            n72 = local read "_HH Channels"() -> (w147:i32[])
            n73 = local read "Config"() -> (w146:T5[])
            n74 = for {
              tunnel: w147 -> [w151] mode=indexing
              shift-right: [w150] -> w145
              shift-left: w146 -> [w152]
              tunnel: w148 -> [w149]
              n75 = in-place {
                in-place-border: w149 -> [w153]
                # "Index / Replace Array Element"
                n76 = in-place-array #1(w152, w151) -> (w155:T5)
                n77 = in-place {
                  in-place-border: w153 -> [w156]
                  n78 = in-place-cluster #2(w155) -> ()  [unwired: 1 out]
                  n79 = in-place-cluster #2("Mode"=w156) -> (w154:T5)
                }
                n80 = in-place-array #1(w154) -> (w150:T5[])  [unwired: 1 out]
              }
            }
            n81 = property on="Config" class="Arr (strict)"("Val(Sgnl)"=w145) -> ()  [unwired: 2 in, 2 out]
          }
          event Value Change {
            n82 = event-data() -> ("NewVal"=w160:bool)  [unwired: 1 out]
            n83 = local read "_HH Channels"() -> (w159:i32[])
            n84 = local read "Config"() -> (w158:T5[])
            n85 = for {
              tunnel: w159 -> [w163] mode=indexing
              shift-right: [w162] -> w157
              shift-left: w158 -> [w164]
              tunnel: w160 -> [w161]
              n86 = in-place {
                in-place-border: w161 -> [w165]
                # "Index / Replace Array Element"
                n87 = in-place-array #3(w164, w163) -> (w167:T5)
                n88 = in-place {
                  in-place-border: w165 -> [w168]
                  n89 = in-place-cluster #4(w167) -> ()  [unwired: 1 out]
                  n90 = in-place-cluster #4("IO Lock State"=w168) -> (w166:T5)
                }
                n91 = in-place-array #3(w166) -> (w162:T5[])  [unwired: 1 out]
              }
            }
            n92 = property on="Config" class="Arr (strict)"("Val(Sgnl)"=w157) -> ()  [unwired: 2 in, 2 out]
          }
          event Value Change {
            n93 = event-data() -> ("NewVal"=w172:bool)  [unwired: 1 out]
            n94 = local read "_HH Channels"() -> (w171:i32[])
            n95 = local read "Config"() -> (w170:T5[])
            n96 = for {
              tunnel: w171 -> [w175] mode=indexing
              shift-right: [w174] -> w169
              shift-left: w170 -> [w176]
              tunnel: w172 -> [w173]
              n97 = in-place {
                in-place-border: w173 -> [w177]
                # "Index / Replace Array Element"
                n98 = in-place-array #5(w176, w175) -> (w179:T5)
                n99 = in-place {
                  in-place-border: w177 -> [w180]
                  n100 = in-place-cluster #6(w179) -> ()  [unwired: 1 out]
                  n101 = in-place-cluster #6("Phase 1 FP"=w180) -> (w178:T5)
                }
                n102 = in-place-array #5(w178) -> (w174:T5[])  [unwired: 1 out]
              }
            }
            n103 = property on="Config" class="Arr (strict)"("Val(Sgnl)"=w169) -> ()  [unwired: 2 in, 2 out]
          }
          event Value Change {
            n104 = event-data() -> ("NewVal"=w184:bool)  [unwired: 1 out]
            n105 = local read "_HH Channels"() -> (w183:i32[])
            n106 = local read "Config"() -> (w182:T5[])
            n107 = for {
              tunnel: w183 -> [w187] mode=indexing
              shift-right: [w186] -> w181
              shift-left: w182 -> [w188]
              tunnel: w184 -> [w185]
              n108 = in-place {
                in-place-border: w185 -> [w189]
                # "Index / Replace Array Element"
                n109 = in-place-array #7(w188, w187) -> (w191:T5)
                n110 = in-place {
                  in-place-border: w189 -> [w192]
                  n111 = in-place-cluster #8(w191) -> ()  [unwired: 1 out]
                  n112 = in-place-cluster #8("Fault Clear"=w192) -> (w190:T5)
                }
                n113 = in-place-array #7(w190) -> (w186:T5[])  [unwired: 1 out]
              }
            }
            n114 = property on="Config" class="Arr (strict)"("Val(Sgnl)"=w181) -> ()  [unwired: 2 in, 2 out]
          }
          event Value Change {
            n115 = event-data() -> ("NewVal"=w196:T7[])  [unwired: 1 out]
            n116 = local read "_HH Channels"() -> (w195:i32[])
            n117 = local read "Config"() -> (w194:T5[])
            n118 = for {
              tunnel: w195 -> [w199] mode=indexing
              shift-right: [w198] -> w193
              shift-left: w194 -> [w200]
              tunnel: w196 -> [w197]
              n119 = in-place {
                in-place-border: w197 -> [w201]
                # "Index / Replace Array Element"
                n120 = in-place-array #9(w200, w199) -> (w203:T5)
                n121 = in-place {
                  in-place-border: w201 -> [w205]
                  n122 = in-place-cluster #10(w203) -> ()  [unwired: 1 out]
                  n123 = Reshape Array(w205, 2 ("dimension size")) -> (w204:T7[])
                  n124 = in-place-cluster #10("ISeq"=w204) -> (w202:T5)
                }
                n125 = in-place-array #9(w202) -> (w198:T5[])  [unwired: 1 out]
              }
            }
            n126 = property on="Config" class="Arr (strict)"("Val(Sgnl)"=w193) -> ()  [unwired: 2 in, 2 out]
          }
          event Value Change {
            n127 = event-data() -> ("NewVal"=w210:T2)  [unwired: 1 out]
            n128 = local read "_HH Channels"() -> (w209:i32[])
            n129 = local read "Command"() -> (w208:T1[])
            n130 = for {
              tunnel: w209 -> [w213] mode=indexing
              shift-right: [w212] -> w207
              shift-left: w208 -> [w214]
              tunnel: w210 -> [w211]
              n131 = in-place {
                in-place-border: w211 -> [w215]
                # "Index / Replace Array Element"
                n132 = in-place-array #11(w214, w213) -> (w217:T1)
                n133 = in-place {
                  in-place-border: w215 -> [w218]
                  n134 = in-place-cluster #12(w217) -> ()  [unwired: 1 out]
                  n135 = in-place-cluster #12("Mode"=w218) -> (w216:T1)
                }
                n136 = in-place-array #11(w216) -> (w212:T1[])  [unwired: 1 out]
              }
            }
            n137 = property on="Command" class="Arr (strict)"("Val(Sgnl)"=w207) -> ()  [unwired: 2 in, 2 out]
          }
          event Value Change {
            n138 = event-data() -> ("NewVal"=w222:T3)  [unwired: 1 out]
            n139 = local read "_HH Channels"() -> (w221:i32[])
            n140 = local read "Command"() -> (w220:T1[])
            n141 = for {
              tunnel: w221 -> [w225] mode=indexing
              shift-right: [w224] -> w219
              shift-left: w220 -> [w226]
              tunnel: w222 -> [w223]
              n142 = in-place {
                in-place-border: w223 -> [w227]
                # "Index / Replace Array Element"
                n143 = in-place-array #13(w226, w225) -> (w229:T1)
                n144 = in-place {
                  in-place-border: w227 -> [w230]
                  n145 = in-place-cluster #14(w229) -> ()  [unwired: 1 out]
                  n146 = in-place-cluster #14("Digital Input"=w230) -> (w228:T1)
                }
                n147 = in-place-array #13(w228) -> (w224:T1[])  [unwired: 1 out]
              }
            }
            n148 = property on="Command" class="Arr (strict)"("Val(Sgnl)"=w219) -> ()  [unwired: 2 in, 2 out]
          }
          event Value Change {
            n149 = event-data() -> ("NewVal"=w234:bool)  [unwired: 1 out]
            n150 = local read "_HH Channels"() -> (w233:i32[])
            n151 = local read "Command"() -> (w232:T1[])
            n152 = for {
              tunnel: w233 -> [w237] mode=indexing
              shift-right: [w236] -> w231
              shift-left: w232 -> [w238]
              tunnel: w234 -> [w235]
              n153 = in-place {
                in-place-border: w235 -> [w239]
                # "Index / Replace Array Element"
                n154 = in-place-array #15(w238, w237) -> (w241:T1)
                n155 = in-place {
                  in-place-border: w239 -> [w242]
                  n156 = in-place-cluster #16(w241) -> ()  [unwired: 1 out]
                  n157 = in-place-cluster #16("Polarity"=w242) -> (w240:T1)
                }
                n158 = in-place-array #15(w240) -> (w236:T1[])  [unwired: 1 out]
              }
            }
            n159 = property on="Command" class="Arr (strict)"("Val(Sgnl)"=w231) -> ()  [unwired: 2 in, 2 out]
          }
          event Value Change {
            n160 = event-data() -> ("NewVal"=w246:sgl)  [unwired: 1 out]
            n161 = local read "_HH Channels"() -> (w245:i32[])
            n162 = local read "Command"() -> (w244:T1[])
            n163 = for {
              tunnel: w245 -> [w249] mode=indexing
              shift-right: [w248] -> w243
              shift-left: w244 -> [w250]
              tunnel: w246 -> [w247]
              n164 = in-place {
                in-place-border: w247 -> [w251]
                # "Index / Replace Array Element"
                n165 = in-place-array #17(w250, w249) -> (w253:T1)
                n166 = in-place {
                  in-place-border: w251 -> [w254]
                  n167 = in-place-cluster #18(w253) -> ()  [unwired: 1 out]
                  n168 = in-place-cluster #18("Frequency [Hz]"=w254) -> (w252:T1)
                }
                n169 = in-place-array #17(w252) -> (w248:T1[])  [unwired: 1 out]
              }
            }
            n170 = property on="Command" class="Arr (strict)"("Val(Sgnl)"=w243) -> ()  [unwired: 2 in, 2 out]
          }
          event Value Change {
            n171 = event-data() -> ("NewVal"=w258:sgl)  [unwired: 1 out]
            n172 = local read "_HH Channels"() -> (w257:i32[])
            n173 = local read "Command"() -> (w256:T1[])
            n174 = for {
              tunnel: w257 -> [w261] mode=indexing
              shift-right: [w260] -> w255
              shift-left: w256 -> [w262]
              tunnel: w258 -> [w259]
              n175 = in-place {
                in-place-border: w259 -> [w263]
                # "Index / Replace Array Element"
                n176 = in-place-array #19(w262, w261) -> (w265:T1)
                n177 = in-place {
                  in-place-border: w263 -> [w266]
                  n178 = in-place-cluster #20(w265) -> ()  [unwired: 1 out]
                  n179 = in-place-cluster #20("Duty Cycle [%]"=w266) -> (w264:T1)
                }
                n180 = in-place-array #19(w264) -> (w260:T1[])  [unwired: 1 out]
              }
            }
            n181 = property on="Command" class="Arr (strict)"("Val(Sgnl)"=w255) -> ()  [unwired: 2 in, 2 out]
          }
          event Value Change {
            n182 = event-data() -> ("NewVal"=w270:sgl)  [unwired: 1 out]
            n183 = local read "_HH Channels"() -> (w269:i32[])
            n184 = local read "Command"() -> (w268:T1[])
            n185 = for {
              tunnel: w269 -> [w273] mode=indexing
              shift-right: [w272] -> w267
              shift-left: w268 -> [w274]
              tunnel: w270 -> [w271]
              n186 = in-place {
                in-place-border: w271 -> [w275]
                # "Index / Replace Array Element"
                n187 = in-place-array #21(w274, w273) -> (w277:T1)
                n188 = in-place {
                  in-place-border: w275 -> [w278]
                  n189 = in-place-cluster #22(w277) -> ()  [unwired: 1 out]
                  n190 = in-place-cluster #22("TDC Offset [CAD]"=w278) -> (w276:T1)
                }
                n191 = in-place-array #21(w276) -> (w272:T1[])  [unwired: 1 out]
              }
            }
            n192 = property on="Command" class="Arr (strict)"("Val(Sgnl)"=w267) -> ()  [unwired: 2 in, 2 out]
          }
          event Value Change {
            n193 = event-data() -> ("NewVal"=w282:sgl)  [unwired: 1 out]
            n194 = local read "_HH Channels"() -> (w281:i32[])
            n195 = local read "Command"() -> (w280:T1[])
            n196 = for {
              tunnel: w281 -> [w285] mode=indexing
              shift-right: [w284] -> w279
              shift-left: w280 -> [w286]
              tunnel: w282 -> [w283]
              n197 = in-place {
                in-place-border: w283 -> [w287]
                # "Index / Replace Array Element"
                n198 = in-place-array #23(w286, w285) -> (w289:T1)
                n199 = in-place {
                  in-place-border: w287 -> [w290]
                  n200 = in-place-cluster #24(w289) -> ()  [unwired: 1 out]
                  n201 = in-place-cluster #24("Window Start [DBTDC]"=w290) -> (w288:T1)
                }
                n202 = in-place-array #23(w288) -> (w284:T1[])  [unwired: 1 out]
              }
            }
            n203 = property on="Command" class="Arr (strict)"("Val(Sgnl)"=w279) -> ()  [unwired: 2 in, 2 out]
          }
          event Value Change {
            n204 = event-data() -> ("NewVal"=w294:sgl)  [unwired: 1 out]
            n205 = local read "_HH Channels"() -> (w293:i32[])
            n206 = local read "Command"() -> (w292:T1[])
            n207 = for {
              tunnel: w293 -> [w297] mode=indexing
              shift-right: [w296] -> w291
              shift-left: w292 -> [w298]
              tunnel: w294 -> [w295]
              n208 = in-place {
                in-place-border: w295 -> [w299]
                # "Index / Replace Array Element"
                n209 = in-place-array #25(w298, w297) -> (w301:T1)
                n210 = in-place {
                  in-place-border: w299 -> [w302]
                  n211 = in-place-cluster #26(w301) -> ()  [unwired: 1 out]
                  n212 = in-place-cluster #26("Window End [DBTDC]"=w302) -> (w300:T1)
                }
                n213 = in-place-array #25(w300) -> (w296:T1[])  [unwired: 1 out]
              }
            }
            n214 = property on="Command" class="Arr (strict)"("Val(Sgnl)"=w291) -> ()  [unwired: 2 in, 2 out]
          }
          event Value Change {
            n215 = event-data() -> ("NewVal"=w306:T4[])  [unwired: 1 out]
            n216 = local read "_HH Channels"() -> (w305:i32[])
            n217 = local read "Command"() -> (w304:T1[])
            n218 = for {
              tunnel: w305 -> [w309] mode=indexing
              shift-right: [w308] -> w303
              shift-left: w304 -> [w310]
              tunnel: w306 -> [w307]
              n219 = in-place {
                in-place-border: w307 -> [w311]
                # "Index / Replace Array Element"
                n220 = in-place-array #27(w310, w309) -> (w313:T1)
                n221 = in-place {
                  in-place-border: w311 -> [w316]
                  n222 = in-place-cluster #28(w313) -> ()  [unwired: 1 out]
                  n223 = Reshape Array(w316, 4 ("dimension size")) -> (w315:T4[])
                  n224 = in-place-cluster #28("Angles"=w315) -> (w312:T1)
                }
                n225 = in-place-array #27(w312) -> (w308:T1[])  [unwired: 1 out]
              }
            }
            n226 = property on="Command" class="Arr (strict)"("Val(Sgnl)"=w303) -> ()  [unwired: 2 in, 2 out]
          }
          event Value Change {
            n227 = event-data() -> ("NewVal"=w320:bool)  [unwired: 1 out]
            n228 = local read "_HH Channels"() -> (w319:i32[])
            n229 = local read "Command"() -> (w318:T1[])
            n230 = for {
              tunnel: w319 -> [w323] mode=indexing
              shift-right: [w322] -> w317
              shift-left: w318 -> [w324]
              tunnel: w320 -> [w321]
              n231 = in-place {
                in-place-border: w321 -> [w325]
                # "Index / Replace Array Element"
                n232 = in-place-array #29(w324, w323) -> (w327:T1)
                n233 = in-place {
                  in-place-border: w325 -> [w328]
                  n234 = in-place-cluster #30(w327) -> ()  [unwired: 1 out]
                  n235 = in-place-cluster #30("Skip Fire"=w328) -> (w326:T1)
                }
                n236 = in-place-array #29(w326) -> (w322:T1[])  [unwired: 1 out]
              }
            }
            n237 = property on="Command" class="Arr (strict)"("Val(Sgnl)"=w317) -> ()  [unwired: 2 in, 2 out]
          }
          event Value Change {
            n238 = event-data() -> ("NewVal"=w332:u8)  [unwired: 1 out]
            n239 = local read "_HH Channels"() -> (w331:i32[])
            n240 = local read "Command"() -> (w330:T1[])
            n241 = for {
              tunnel: w331 -> [w335] mode=indexing
              shift-right: [w334] -> w329
              shift-left: w330 -> [w336]
              tunnel: w332 -> [w333]
              n242 = in-place {
                in-place-border: w333 -> [w337]
                # "Index / Replace Array Element"
                n243 = in-place-array #31(w336, w335) -> (w339:T1)
                n244 = in-place {
                  in-place-border: w337 -> [w340]
                  n245 = in-place-cluster #32(w339) -> ()  [unwired: 1 out]
                  n246 = in-place-cluster #32("Skip Fire Index"=w340) -> (w338:T1)
                }
                n247 = in-place-array #31(w338) -> (w334:T1[])  [unwired: 1 out]
              }
            }
            n248 = property on="Command" class="Arr (strict)"("Val(Sgnl)"=w329) -> ()  [unwired: 2 in, 2 out]
          }
          event "_HH Channels": Value Change {
            n249 = event-data() -> ()  [unwired: 7 out]
            n250 = property on="_Refresh" class="Bool (strict)"("Val(Sgnl)"=TRUE ("Value (Signaling)")) -> ()  [unwired: 2 in, 2 out]
          }
          event "_Refresh": Value Change {
            n251 = event-data() -> ()  [unwired: 7 out]
            n252 = local write "_Refresh"(FALSE ("_Refresh")) -> ()
            n253 = stacked-sequence {
              frame #0 {
                n254 = local read "_HH Channels"() -> (w345:i32[])
                n255 = local read "Channel Names"() -> (w346:string[])
                n256 = local read "Command"() -> (w350:T1[])
                n257 = local read "Config"() -> (w351:T5[])
                n258 = Index Array(array=w345, index=0) -> (element=w344:i32)
                n259 = Index Array(array=w351, index=w344) -> (element=w348:T5)
                n260 = Index Array(array=w350, index=w344) -> (element=w349:T1)
                n261 = Index Array(array=w346, index=w344) -> (element=w347:string)
                n262 = local write "_CommandElement"(w349) -> ()
                n263 = local write "Channel Name"(w347) -> ()
                n264 = local write "_ConfigElement"(w348) -> ()
              }
              frame #1 {
                n265 = control-ref of="_HH Channels"() -> (w352:refnum<vi>)
                n266 = local read "Channel Names"() -> (w354:string[])
                n267 = local read "Command"() -> (w353:T1[])
                n268 = local read "Config"() -> (w355:T5[])
                n269 = call "Refresh HH Listbox.vi"("Command"=w353, "Names"=w354, "Config"=w355, "_Listbox"=w352) -> ()  [unwired: 6 in, 2 out]
              }
            }
          }
        }
        n270 = call <vilib>:"Simple Error Handler.vi"("error in (no error)"=w65) -> ("error out"=w64:errorcluster)  [unwired: 1 in, 7 out]
        n271 = call <vilib>:"Clear Errors.vi"("error in (no error)"=w64) -> ("error out"=w63:errorcluster)  [unwired: 1 in, 5 out]
      }
      n272 = Unregister For Events(event registration refnum=w61, error in=w60) -> (error out=w59:errorcluster)
    }
    frame Error {
      n273 = call <vilib>:"Simple Error Handler.vi"("error in (no error)"=w358) -> ("error out"=w357:errorcluster)  [unwired: 1 in, 7 out]
      n274 = call <vilib>:"Clear Errors.vi"("error in (no error)"=w357) -> ("error out"=w356:errorcluster)  [unwired: 1 in, 5 out]
    }
  }
  n275 = invoke class="VI" method="FP.Close"(error in=w12) -> (error out=w11:errorcluster)  [unwired: 2 in, 2 out]
  n276 = call <vilib>:"NI VeriStand - Signal When Ready for Shutdown.vi"("error in (no error)"=w11) -> ("error out"=→"error out":errorcluster)  [unwired: 10 out]
